vi "Load ANI Textures.vi"(6 "Scale":sgl=1.0, 7 "Renderer":u32, 8 "error in (no error)":errorcluster, 11 "Path":path) -> (0 "error out":errorcluster, 2 "Hotspots":refnum<class "Vector 2D.lvclass">[](array[class]), 3 "Names":string[](array[string]))   [LabVIEW 2021]
uses:
  Re-use Libraries/Vector 2D/Vector 2D.lvclass
  <userlib>/_OpenG.lib/string/string.llb/openg_string.lvlib
  Resource Manager/Resource Manager.lvclass
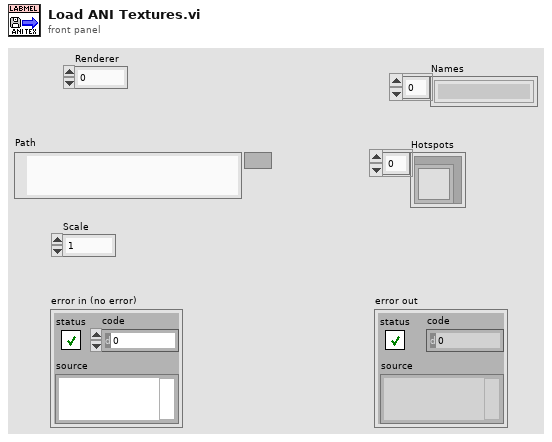
[diagram p1: front panel]
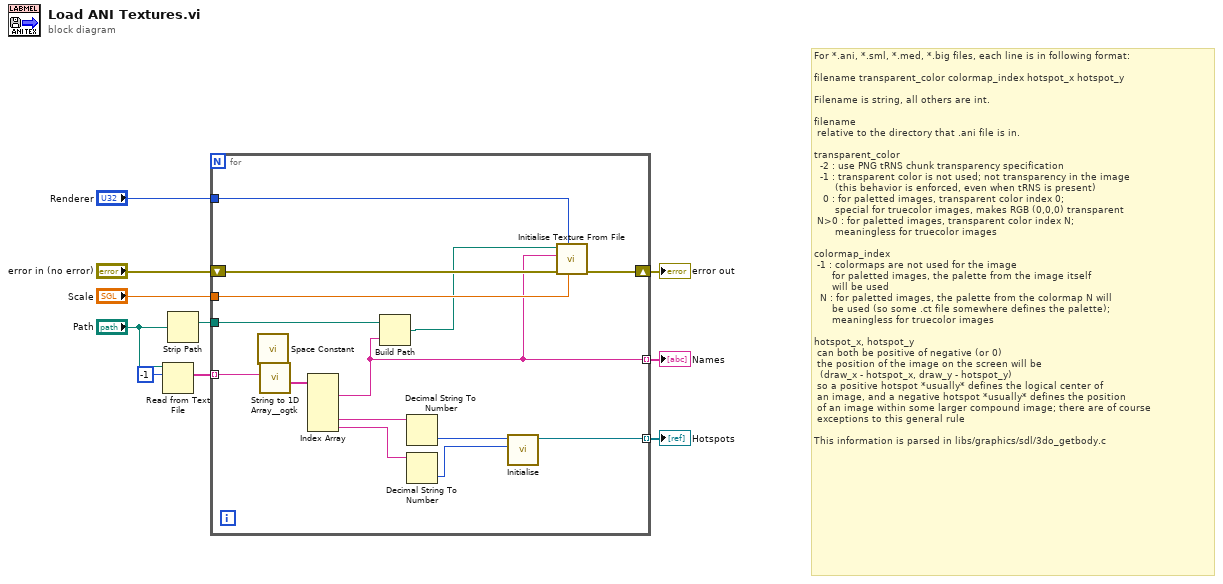
[diagram p0: block diagram]
diagram:
  # "For *.ani, *.sml, *.med, *.big files, each line is in following format:\n\nfilename transparent_color colormap_index hotspot_x hotspot_y\n\nFilename is string, all others are int.\n\nfilename\n\trelative to the directory that .ani file is in.\n\ntransparent_color\n\t -2 : use PNG tRNS chunk transparency specification\n\t -1 : transparent color is not used; not transparency in the image\n\t      (this behavior is enforced, even when tRNS is present)\n\t  0 : for paletted images, transparent color index 0;\n\t      special for truecolor images, makes RGB (0,0,0) transparent\n\tN>0 : for paletted images, transparent color index N;\n\t      meaningless for truecolor images\n\ncolormap_index\n\t-1 : colormaps are not used for the image\n\t     for paletted images, the palette from the image itself\n\t     will be used\n\t N : for paletted images, the palette from the colormap N will\n\t     be used (so some .ct file somewhere defines the palette);\n\t     meaningless for truecolor images\n\nhotspot_x, hotspot_y\n\tcan both be positive of negative (or 0)\n\tthe position of the image on the screen will be\n\t\t(draw_x - hotspot_x, draw_y - hotspot_y)\n\tso a positive hotspot *usually* defines the logical center of\n\tan image, and a negative hotspot *usually* defines the position\n\tof an image within some larger compound image; there are of course\n\texceptions to this general rule\n\nThis information is parsed in libs/graphics/sdl/3do_getbody.c"
  n1 = Read from Text File(file (use dialog)="Path", count=-1) -> (text=w8:string[])  [unwired: 2 in, 3 out]
  n2 = Strip Path(path="Path") -> (stripped path=w7:path)  [unwired: 1 out]
  n3 = for {
    tunnel: w8 -> [w20] mode=indexing
    tunnel: w7 -> [w21]
    tunnel: [w11] -> w6 mode=indexing
    tunnel: "Scale" -> [w17]
    shift-right: [w18] -> w3
    shift-left: "error in (no error)" -> [w19]
    tunnel: [w15] -> w2 mode=indexing
    tunnel: "Renderer" -> [w14]
    n4 = call <vilib>:"Space Constant.vi"() -> ("String"=w22:string)
    n5 = call <userlib>:"String to 1D Array__ogtk.vi"("delimiter (Tab)"=w22, "string"=w20) -> ("Array of Strings"=w23:string[])  [unwired: 9 in]
    n6 = Index Array(array=w23) -> (element #1=w15:string, element #4=w24:string, element #5=w25:string)  [unwired: 5 in, 2 out]
    n7 = Build Path(base path=w21, name or relative path=w15) -> (appended path=w16:path)
    n8 = Decimal String To Number(string=w24) -> (number=w13:i32)  [unwired: 2 in, 1 out]
    n9 = Decimal String To Number(string=w25) -> (number=w12:i32)  [unwired: 2 in, 1 out]
    n10 = call "Initialise.vi"("y"=w12, "x"=w13) -> ("Vector 2D out"=w11:refnum<class "Vector 2D.lvclass">)  [unwired: 9 in]
    n11 = call "Initialise Texture From File.vi"("Scale"=w17, "Renderer"=w14, "error in (no error)"=w19, "Name"=w15, "File"=w16) -> ("error out"=w18:errorcluster)  [unwired: 5 in, 1 out]
  }
  "error out" <- w3
  "Hotspots" <- w6
  "Names" <- w2
